vi "read_basic_log.vi"() -> ()   [LabVIEW 2013]
uses:
  cRIO_Code/Data/TypeDefs/Notifiers.ctl
  cRIO_Code/Data/TypeDefs/UTM Location.ctl
  cRIO_Code/Data/TypeDefs/Sail Set Suggestions.ctl
  cRIO_Code/Data/TypeDefs/Rudder Set Suggestions.ctl
  cRIO_Code/Data/TypeDefs/OverrideInformation.ctl
  cRIO_Code/Data/TypeDefs/OverrideMode.ctl
  cRIO_Code/Data/TypeDefs/MotorSetup.ctl
  cRIO_Code/Data/TypeDefs/DynamixelSetupInfo.ctl
  cRIO_Code/Data/TypeDefs/AirmarStatus.ctl
  cRIO_Code/Data/TypeDefs/HardwareOnline.ctl
  cRIO_Code/Data/TypeDefs/DynamixelCycleTracker.ctl
  cRIO_Code/Data/TypeDefs/RC Input Values.ctl
  cRIO_Code/Logic/Classes/Waypoint/Waypoint.lvclass
panel:
  out "size(s)":i32
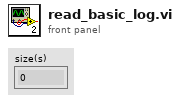
[diagram p1: front panel]
types:
  T1 = typedef "Notifiers.ctl" = cluster{"BoatSpeed":refnum<notifier>, "WindSpeed":refnum<notifier>, "EStop":refnum<notifier>, "BoatDirection":refnum<notifier>, "Luffing":refnum<notifier>, "RudderForce":refnum<notifier>, "BatteryVoltage":refnum<notifier>, "StayForces":refnum<notifier>, "BoatLocation":refnum<notifier>, "Pitch":refnum<notifier>, "Roll":refnum<notifier>, "RateOfTurn":refnum<notifier>, "RelWindDirection":refnum<notifier>, "SailPositions":refnum<notifier>, "RudderPosition":refnum<notifier>, "IronsRange":refnum<notifier>, "AbsWindDirection":refnum<notifier>, "OverrideInformation":refnum<notifier>, "DynamixelTorques":refnum<notifier>, "MotorSetup":refnum<notifier>, "AirmarStatus":refnum<notifier>, "HardwareOnline?":refnum<notifier>, "Sim_ActualSailPositions [0,1]":refnum<notifier>, "DynamixelCycleTracker":refnum<notifier>, "BoatVelocityDirection":refnum<notifier>, "SimWindHeading(rad)":refnum<notifier>, "SimWindSpeed(m/s)":refnum<notifier>, "RCInputValues":refnum<notifier>, "Finished Waypoints":refnum<notifier>, "DesiredHeading":refnum<notifier>, "Latest Mission ID":refnum<notifier>, "Latest Obstacle ID":refnum<notifier>, "DownwindDiscouragedRange":refnum<notifier>, "Tack Range":refnum<notifier>}
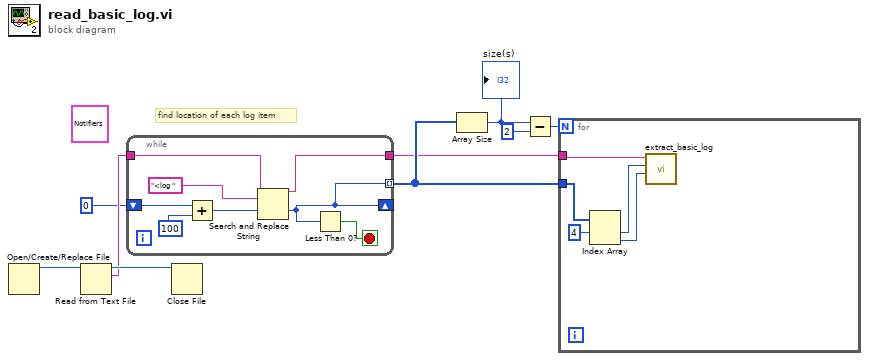
[diagram p0: block diagram]
diagram:
  (unwired) T1 {"BoatSpeed"=refnum, "WindSpeed"=refnum, "EStop"=refnum, "BoatDirection"=refnum, "Luffing"=refnum, "RudderForce"=refnum, "BatteryVoltage"=refnum, "StayForces"=refnum, "BoatLocation"=refnum, "Pitch"=refnum, "Roll"=refnum, "RateOfTurn"=refnum, "RelWindDirection"=refnum, "SailPositions"=refnum, "RudderPosition"=refnum, "IronsRange"=refnum, "AbsWindDirection"=refnum, "OverrideInformation"=refnum, "DynamixelTorques"=refnum, "MotorSetup"=refnum, "AirmarStatus"=refnum, "HardwareOnline?"=refnum, "Sim_ActualSailPositions [0,1]"=refnum, "DynamixelCycleTracker"=refnum, "BoatVelocityDirection"=refnum, "SimWindHeading(rad)"=refnum, "SimWindSpeed(m/s)"=refnum, "RCInputValues"=refnum, "Finished Waypoints"=refnum, "DesiredHeading"=refnum, "Latest Mission ID"=refnum, "Latest Obstacle ID"=refnum, "DownwindDiscouragedRange"=refnum, "Tack Range"=refnum} ("NotifierReferences")
  # "find location of each log item"
  n1 = Open/Create/Replace File() -> (refnum out=w9:refnum<file>)  [unwired: 6 in, 2 out]
  n2 = Read from Text File(file (use dialog)=w9) -> (refnum out=w8:refnum<file>, text=w7:string)  [unwired: 3 in, 2 out]
  n3 = while {
    tunnel: w7 -> [w17]
    shift-right: [w10] -> _
    shift-left: 0 ("offset past replacement") -> [w14]
    tunnel: [w11] -> w1
    tunnel: [w10] -> w2 mode=indexing
    stop <- w15 stop-if-true
    n4 = Add(x=w14, y=100) -> (x+y=w13:i32)
    n5 = Search and Replace String(input string=w17, search string="<log ", offset=w13) -> (result string=w11:string, offset past replacement=w10:i32)  [unwired: 5 in, 2 out]
    n6 = Less Than 0?(x=w10) -> (x < 0?=w15:bool)
  }
  n7 = Close File(refnum=w8) -> ()  [unwired: 1 in, 2 out]
  n8 = Array Size(array=w2) -> (size(s)=w5:i32)
  "size(s)" <- w5
  n9 = Subtract(x=w5, y=2) -> (x-y=w3:i32)
  n10 = for {
    N: w3 -> [_]
    tunnel: w2 -> [w22]
    tunnel: w1 -> [w20]
    n11 = Index Array(array=w22, index #1=4 ("index")) -> (element #1=w19:i32, element #2=w18:i32)  [unwired: 1 in]
    n12 = call "extract_basic_log.vi"("Next element index"=w18, "Current element index"=w19, "total string"=w20) -> ()  [unwired: 9 in]
  }
